vi "Module Template State Machine.vi"() -> ()   [LabVIEW 2019]
panel:
  out "length 3":i32
  out "length 2":i32
  out "length":i32
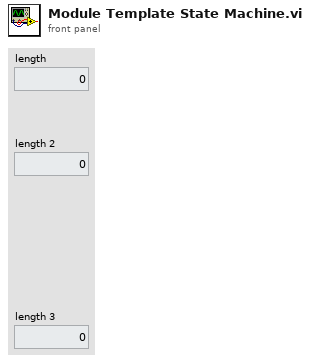
[diagram p1: front panel]
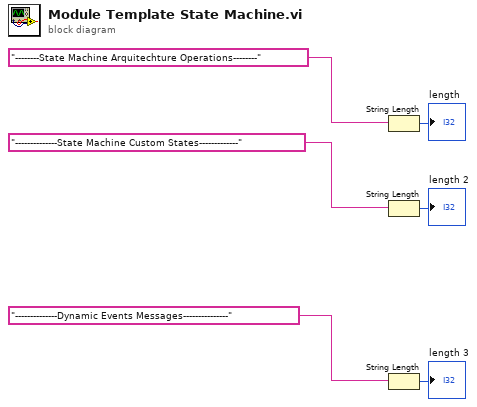
[diagram p0: block diagram]
diagram:
  n1 = String Length(string="--------State Machine Arquitechture Operations--------") -> (length=→"length":i32)
  n2 = String Length(string="--------------State Machine Custom States-------------") -> (length=→"length 2":i32)
  n3 = String Length(string="--------------Dynamic Events Messages---------------") -> (length=→"length 3":i32)
